vi "Main.vi"(10 "Tree Ref":refnum<vi>, 11 "Module Admin":refnum<class "Delacor_lib_QMH_Cloneable Module Admin.lvclass">) -> ()   [LabVIEW 2023, in "Tree Handlr.lvlib"]
doc: "This template is based off of the Queued Message Handler design pattern and the Queued Message Handler project template that ships with LabVIEW.\n\nThe main difference is that the queue is private to this module and communication between modules is performed via Broadcast and Request events.\n\nRequest events are wrapped in public API methods and are handled in the Event Handling Loop (EHL) of this VI. Any module can register for Broadcast events sent by this module. The EHL generates messages based on user interface actions.\n\nThe Message Handling Loop (MHL) processes messages generated by the EHL, or by other messages. The messages are string values, so new messages can be added easily to the Message Cases case structure in the MHL. Each message cluster can also provide an optional value for Message Data, which is a variant that can be converted to whatever message-specific data is required.\n_____\nBased on DQMH Project Template 7.0.1.1316."
uses:
  Tree Handlr.lvlib
  <vilib>/Delacor/Delacor QMH/Libraries/Cloneable Module Admin_class/Delacor_lib_QMH_Cloneable Module Admin.lvclass
  Module Data--cluster.ctl
  <vilib>/Delacor/Delacor QMH/Libraries/Message Queue_class/Delacor_lib_QMH_Message Queue.lvclass/Delacor_lib_QMH_Message Queue.ctl
  <vilib>/Delacor/Delacor QMH/Libraries/Cloneable Module Admin_class/Delacor_lib_QMH_Cloneable Module Admin.lvclass/Delacor_lib_QMH_Cloneable Module Admin.ctl
  Stop Argument--cluster.ctl
  <vilib>/Delacor/Delacor QMH/Libraries/Module Admin_class/Delacor_lib_QMH_Module Admin.lvclass/Delacor_lib_QMH_Module Admin.ctl
  Restore Open Items Argument--cluster.ctl
  <vilib>/Utility/miscctls.llb/LVPointTypeDef.ctl
  <vilib>/Delacor/Delacor QMH/Libraries/Message Queue_class/Delacor_lib_QMH_Enqueue Message (Multiline).vi
  <vilib>/Delacor/Delacor QMH/Libraries/Cloneable Module Admin_class/Delacor_lib_QMH_Get Module ID.vi
  <vilib>/Delacor/Delacor QMH/Libraries/Module Admin_class/Delacor_lib_QMH_Get External Launch.vi
  LabVIEW-common/TEMPLATES/State Machine/State Machine Sub/Process Multi-LineState String.vi
  <vilib>/Utility/inputDevices.llb/keyboardAcquire.vi
  <vilib>/Delacor/Delacor QMH/Libraries/Message Queue_class/Delacor_lib_QMH_Message Queue.lvclass
panel:
  out "error out":errorcluster
  out "Status":string
  in  "Simulate EHL Error":bool
  in  "Simulate MHL Error":bool
  # "Other processes communicate with this Module via its Public API (wrappers for its Request Events).\n\nThis Module communicates with other processes via its Broadcast Events.\nAny process that wants to receive these messages can register for this module's Broadcast events."
  # "This template is for the DQMH framework. See the block diagram for more information on how to use this template."
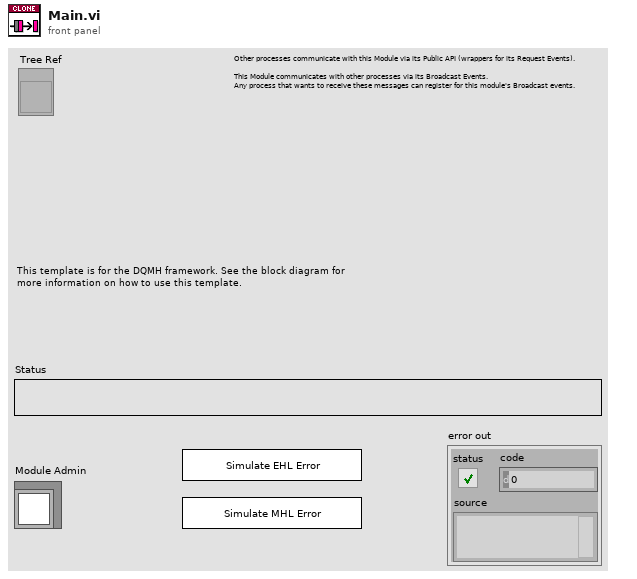
[diagram p1: front panel]
types:
  T1 = typedef "Tree Handlr.lvlib/Request Events--cluster.ctl" = cluster{"Stop Module":refnum<user-event>, "Show Panel":refnum<user-event>, "Hide Panel":refnum<user-event>, "Show Diagram":refnum<user-event>, "Get Module Execution Status":refnum<user-event>, "Restore Open Items":refnum<user-event>}
  T2 = typedef "Tree Handlr.lvlib/Module Data--cluster.ctl" = cluster{"Status":string}
  T3 = enum32{"invalid lock state", "Not Locked", "Locked (No Password)", "Password-protected"}
  T4 = typedef "Tree Handlr.lvlib/Stop Argument--cluster.ctl" = cluster{"Module ID":i32, "Origin":string, "Exit via Stop Module Req?":bool, "Wait for Module to stop?":bool}
  T5 = enum16{"0", "1", "2", "3", "4", "5", "6", "7", "8", "9", "A", "B", "C", "D", "E", "F", "G", "H", "I", "J", "K", "L", "M", "N", "O", "P", "Q", "R", "S", "T", "U", "V", "W", "X", "Y", "Z", "F1", "F2", "F3", "F4", "F5", "F6", "F7", "F8", "F9", "F10", "F11", "F12", "F13", "F14", "F15", "ADD", "BACK", "BACKSLASH", "CAPITAL", "COMMA", "DECIMAL", "DELETE", "DIVIDE", "DOWN", "END", "EQUALS", "ESCAPE", "GRAVE (`)", "HOME", "INSERT", "LBRACKET", "LCONTROL", "LEFT", "L ALT", "LSHIFT", "LWIN", "MINUS", "MULTIPLY", "NEXT", "NUMLOCK", "NUMPAD_0", "NUMPAD_1", "NUMPAD_2", "NUMPAD_3", "NUMPAD_4", "NUMPAD_5", "NUMPAD_6", "NUMPAD_7", "NUMPAD_8", "NUMPAD_9", "PAUSE", "PERIOD", "PRIOR (PG UP)", "RBRACKET", "RCONTROL", "RETURN", "RIGHT", "R ALT", "RSHIFT", "RWIN", "SCROLL", "SEMICOLON", "SLASH", "SPACE", "SUBTRACT", "TAB", "UP", "ENTER (num pad)", "' (quote)"}
  T6 = typedef "Tree Handlr.lvlib/Restore Open Items Argument--cluster.ctl" = cluster{"Module ID":i32, "Boolean":bool}
  T7 = typedef "LVPointTypeDef.ctl" = cluster{"Horizontal":i16, "Vertical":i16}
  T8 = enum32{"Invalid", "Standard", "Closed", "Hidden", "Minimized", "Maximized"}
  T9 = enum16{"0", "1", "2", "3", "4", "5", "6", "7", "8", "9", "A", "B", "C", "D", "E", "F", "G", "H", "I", "J", "K", "L", "M", "N", "O", "P", "Q", "R", "S", "T", "U", "V", "W", "X", "Y", "Z", "F1", "F2", "F3", "F4", "F5", "F6", "F7", "F8", "F9", "F10", "F11", "F12", "F13", "F14", "F15", "ADD", "BACK", "BACKSLASH", "CAPITAL", "COMMA", "DECIMAL", "DELETE", "DIVIDE", "DOWN", "END", "EQUALS", "ESCAPE", "GRAVE (`)", "HOME", "INSERT", "LBRACKET", "LCONTROL", "LEFT", "L ALT", "LSHIFT", "LWIN", "MINUS", "MULTIPLY", "NEXT", "NUMLOCK", "NUMPAD_0", "NUMPAD_1", "NUMPAD_2", "NUMPAD_3", "NUMPAD_4", "NUMPAD_5", "NUMPAD_6", "NUMPAD_7", "NUMPAD_8", "NUMPAD_9", "PAUSE", "PERIOD", "PRIOR (PG UP)", "RBRACKET", "RCONTROL", "RETURN", "RIGHT", "R ALT", "RSHIFT", "RWIN", "SCROLL", "SEMICOLON", "SLASH", "SPACE", "SUBTRACT", "TAB", "UP", "ENTER (num pad)", "' (quote)"}[]
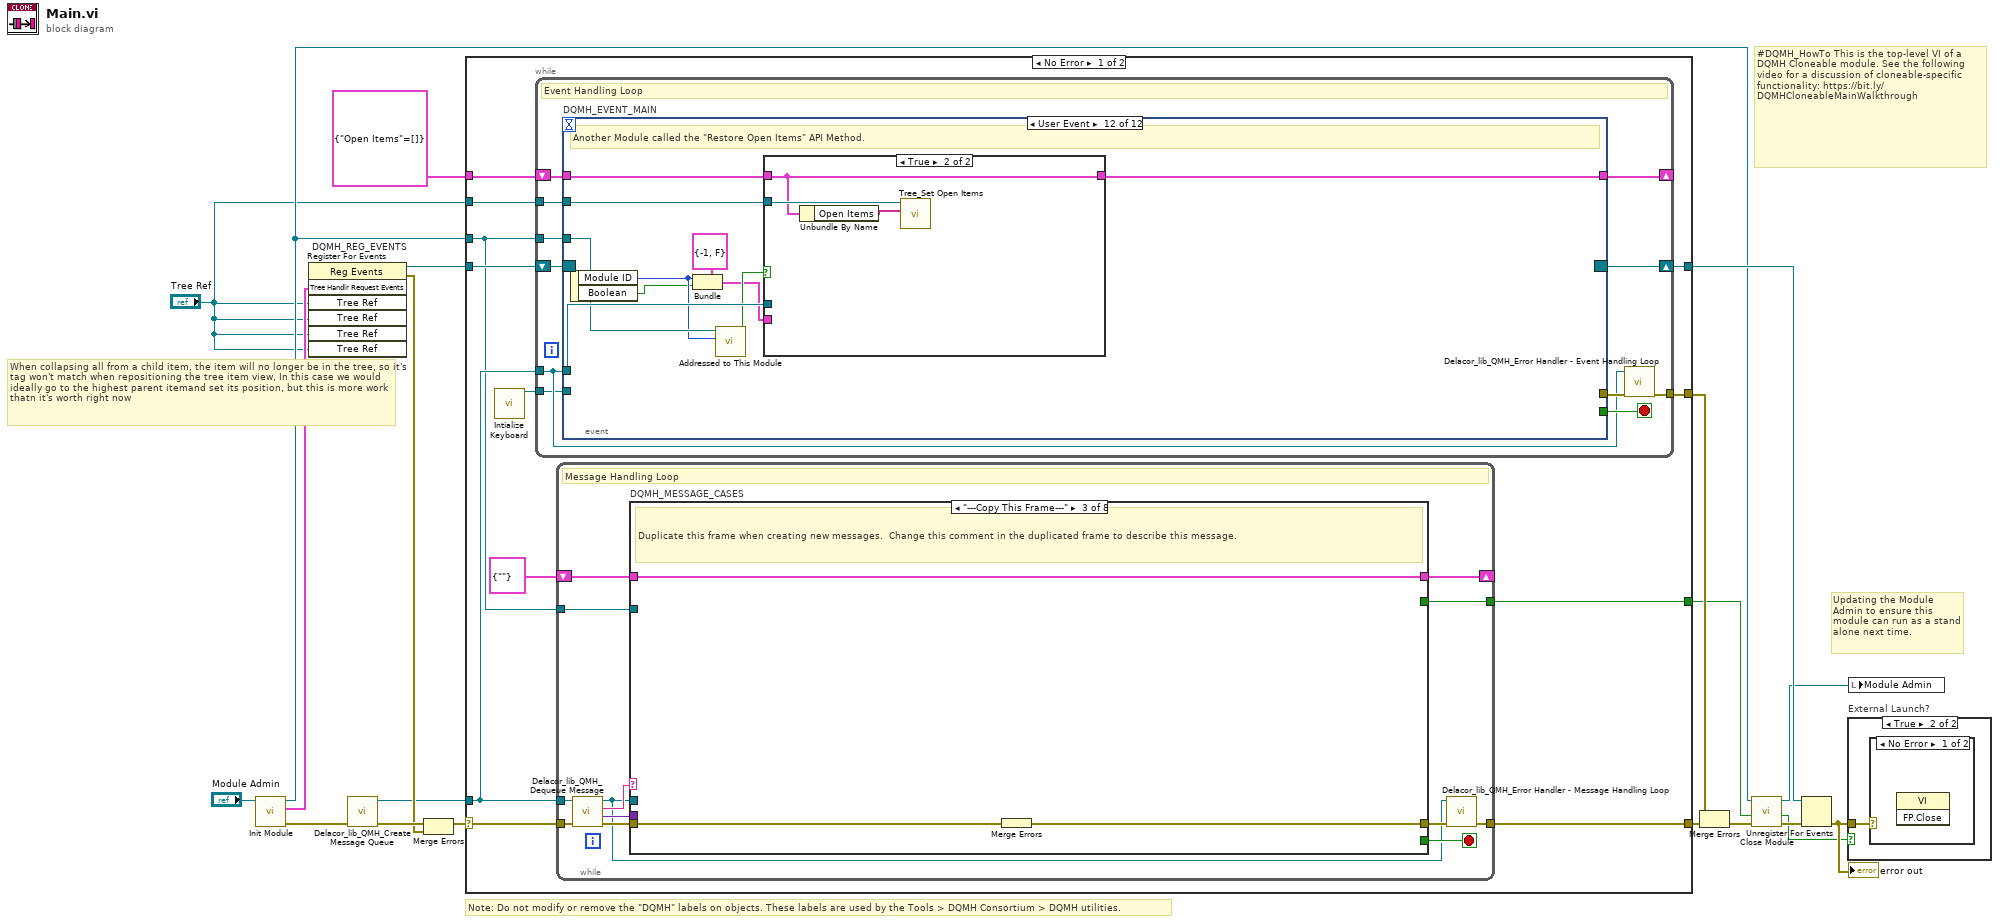
[diagram p0: block diagram]
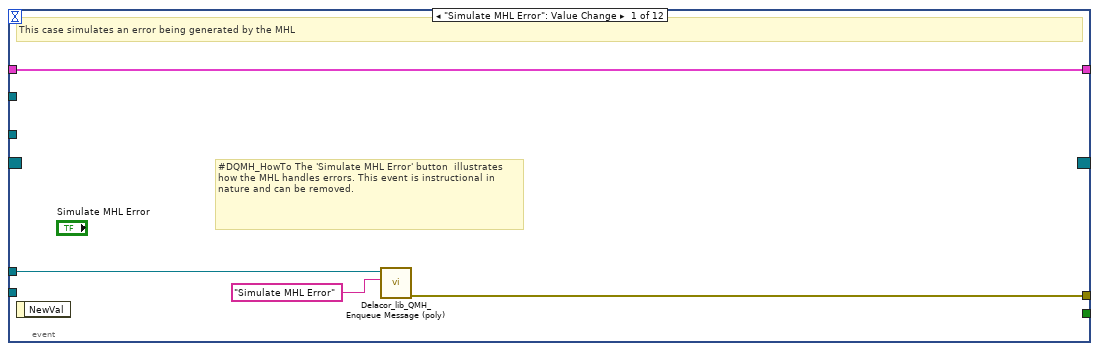
[diagram p2: hidden frame]
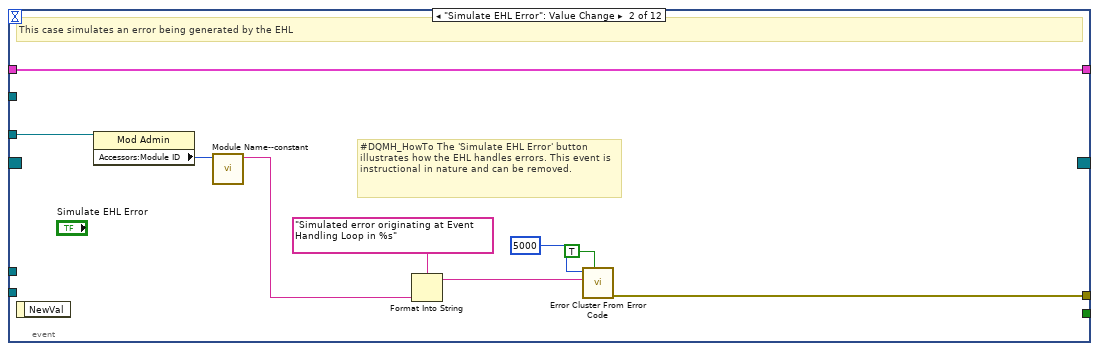
[diagram p3: hidden frame]
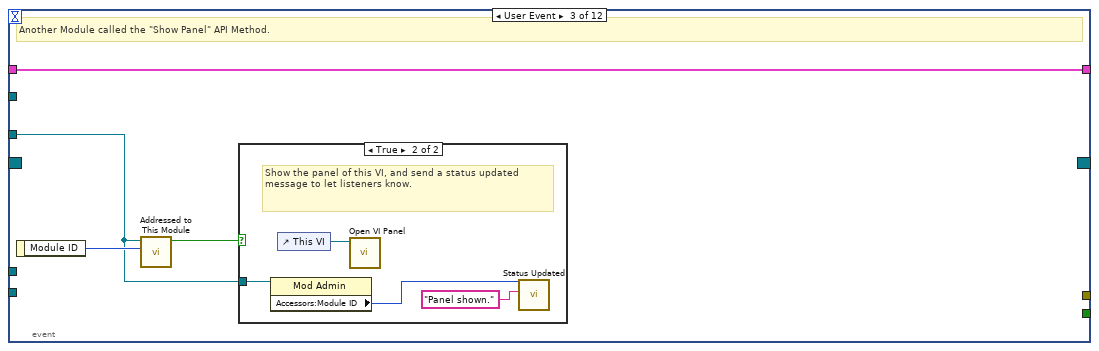
[diagram p4: hidden frame]
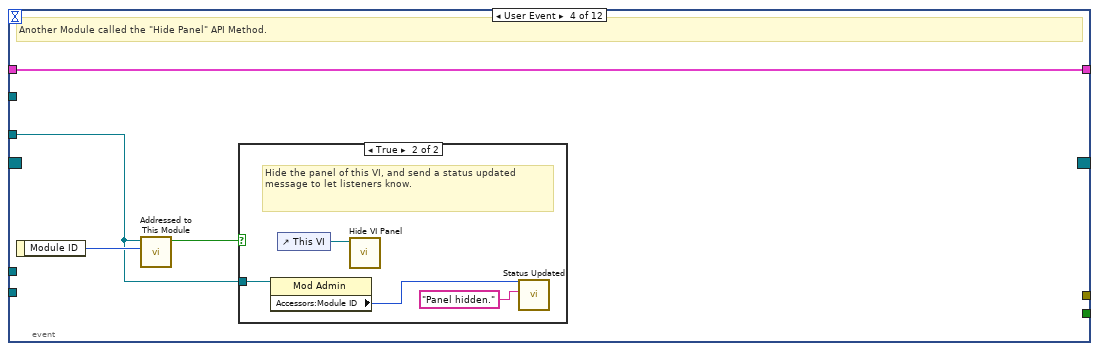
[diagram p6: hidden frame]
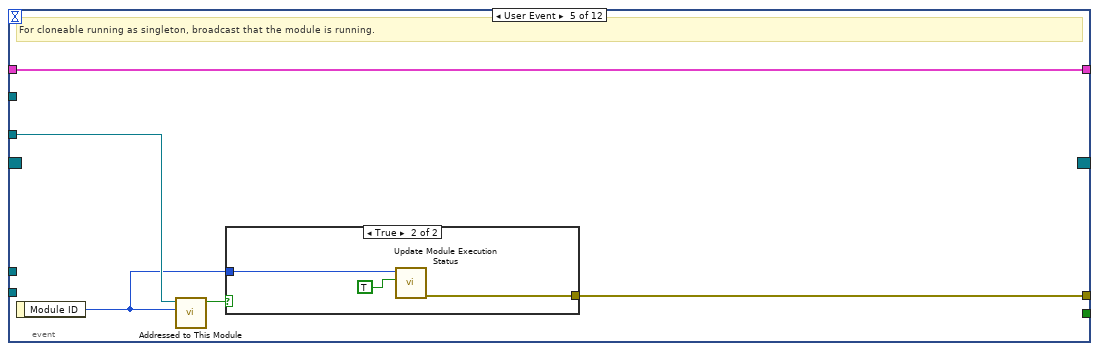
[diagram p8: hidden frame]
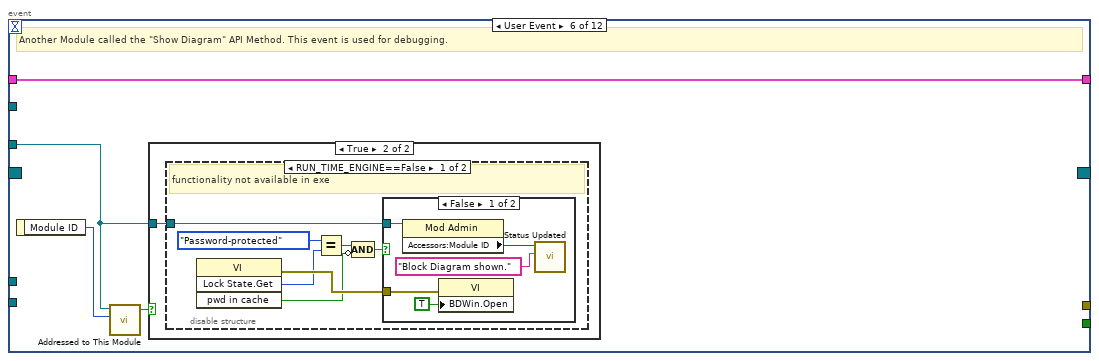
[diagram p10: hidden frame]
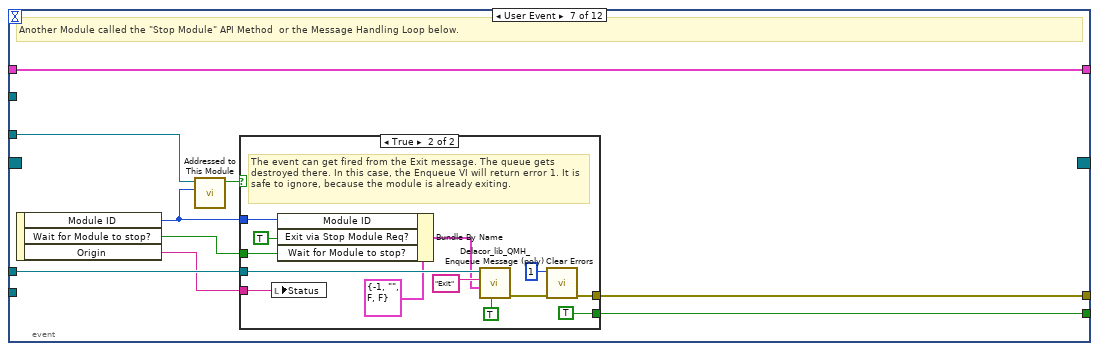
[diagram p14: hidden frame]
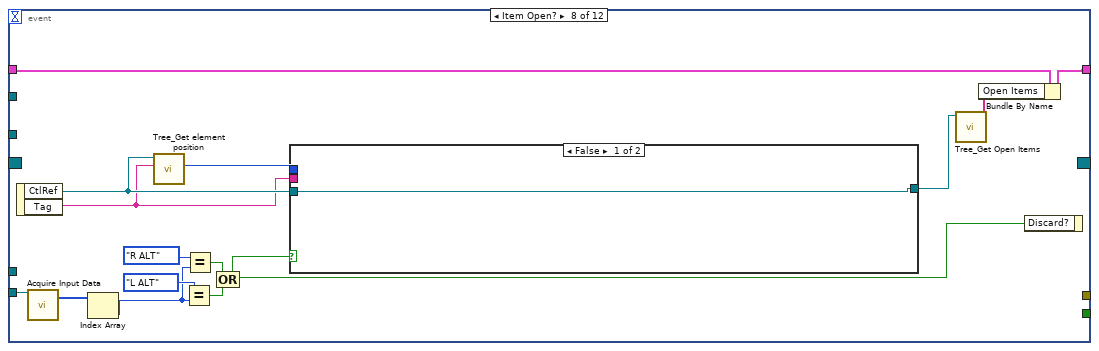
[diagram p16: hidden frame]
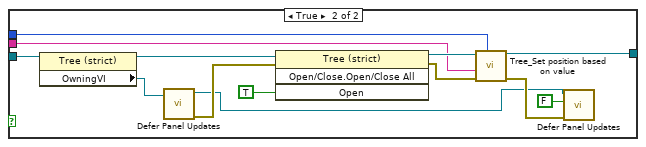
[diagram p17: hidden frame]
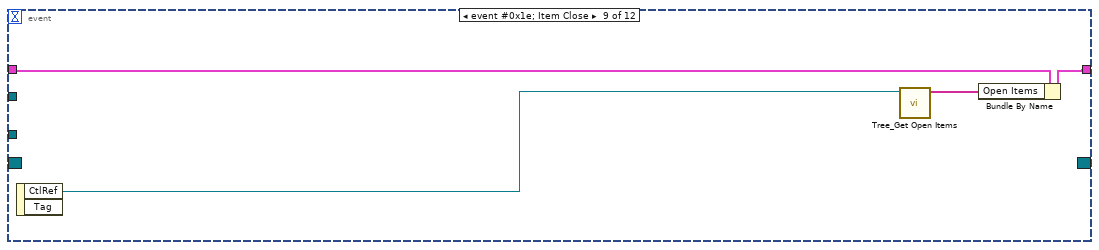
[diagram p18: hidden frame]
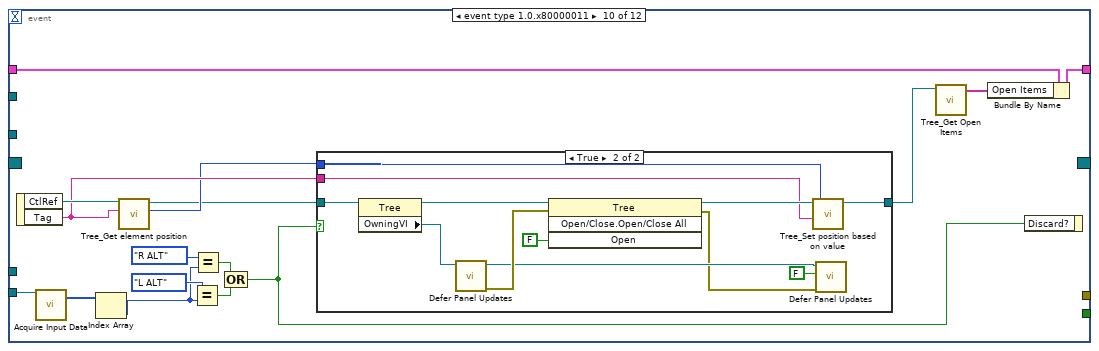
[diagram p19: hidden frame]
diagram:
  # "When collapsing all from a child item, the item will no longer be in the tree, so it's tag won't match when repositioning the tree item view, In this case we would ideally go to the highest parent itemand set its position, but this is more work thatn it's worth right now"
  # "#DQMH_HowTo This is the top-level VI of a DQMH Cloneable module. See the following video for a discussion of cloneable-specific functionality: https://bit.ly/DQMHCloneableMainWalkthrough"
  # "Note: Do not modify or remove the \"DQMH\" labels on objects. These labels are used by the Tools > DQMH Consortium > DQMH utilities."
  # "Updating the Module Admin to ensure this module can run as a stand alone next time."
  n1 = call "Init Module.vi"("Cloneable Module Admin in"="Module Admin") -> ("error out"=w17:errorcluster, "Tree Handlr Request Events"=w9:T1, "Cloneable Module Admin out"=w6:refnum<class "Delacor_lib_QMH_Cloneable Module Admin.lvclass">)  [unwired: 8 in]
  n2 = register-events "DQMH_REG_EVENTS"(w9, "Tree Ref", "Tree Ref", "Tree Ref", "Tree Ref") -> (reference out=w10:refnum<event-registration>, error out=w12:errorcluster)  [unwired: 2 in]
  n3 = call <vilib>:"Delacor_lib_QMH_Create Message Queue.vi"("error in"=w17) -> ("error out"=w14:errorcluster, "Message Queue"=w8:refnum<class "Delacor_lib_QMH_Message Queue.lvclass">)  [unwired: 9 in]
  n4 = Merge Errors(w14, w12) -> (w13:errorcluster)
  n5 = case shown="No Error" w13 {
    selector: w13 -> [w30 w320]
    tunnel: [w32 w319] -> w18
    tunnel: [w29 w318] -> w11
    tunnel: w10 -> [w27 w318]
    tunnel: w8 -> [w26 w311]
    tunnel: [w31 _] -> w19
    tunnel: w6 -> [w25 w314]
    tunnel: [w24 _] -> w4
    tunnel: cluster{"Open Items":string[]} {"Open Items"=[]} -> [w22 _]
    tunnel: "Tree Ref" -> [w21 _]
    frame No Error {
      n6 = call <vilib>:"Intialize Keyboard.vi"() -> ("device ID"=w23:refnum<k1>)  [unwired: 10 in, 1 out]
      n7 = while {
        tunnel: w26 -> [w37]
        shift-right: [w40] -> w29
        shift-left: w27 -> [w41]
        tunnel: [w42] -> w31
        tunnel: w25 -> [w38]
        tunnel: w23 -> [w36]
        shift-right: [w34] -> _
        shift-left: w22 -> [w35]
        tunnel: w21 -> [w33]
        stop <- w39 stop-if-true
        # "Event Handling Loop"
        n8 = event "DQMH_EVENT_MAIN" shown="[8] <Tree Ref>: Item Open;  <Tree Ref>: Item Close" {
          selector: w41 -> [_ _ _ _ _ _ _ _ _ _ _ _]
          dyn-events: [_ _ _ _ _ _ _ _ _ _ _ _] -> w40
          timeout: _ -> [_ _ _ _ _ _ _ _ _ _ _ _]
          tunnel: [_ _ _ _ _ _ w102 _ _ _ _ _] -> w39
          tunnel: w37 -> [w46 _ _ _ _ _ w105 _ _ _ w185 w207]
          tunnel: [w47 w56 _ _ w77 _ w106 _ _ _ w188 _] -> w43
          tunnel: w38 -> [_ w55 w58 w66 w75 w82 w104 _ _ _ w186 w205]
          tunnel: w36 -> [_ _ _ _ _ _ _ w128 _ w162 _ _]
          tunnel: w35 -> [w44 w48 w57 w65 w73 w81 w98 w123 w152 w157 w182 w199]
          tunnel: [w44 w48 w57 w65 w73 w81 w98 w122 w151 w156 w182 w198] -> w34
          tunnel: w33 -> [_ _ _ _ _ _ _ _ _ _ _ w200]
          event "Simulate MHL Error": Value Change {
            # "#DQMH_HowTo The 'Simulate MHL Error' button  illustrates how the MHL handles errors. This event is instructional in nature and can be removed."
            # "This case simulates an error being generated by the MHL"
            n9 = event-data() -> ()  [unwired: 1 in, 1 out]
            n10 = call-poly <vilib>:"Delacor_lib_QMH_Enqueue Message (poly).vi"("Message"="Simulate MHL Error", "Message Queue in"=w46) -> ("error out"=w47:errorcluster)  [unwired: 8 in, 1 out]
          }
          event "Simulate EHL Error": Value Change {
            # "#DQMH_HowTo The 'Simulate EHL Error' button  illustrates how the EHL handles errors. This event is instructional in nature and can be removed."
            # "This case simulates an error being generated by the EHL"
            n11 = event-data() -> ()  [unwired: 1 in, 1 out]
            n12 = property on="Property Node" class="Mod Admin"(reference=w55) -> ("Accessors:Module ID"=w54:i32)  [unwired: 1 in, 2 out]
            n13 = call "Module Name--constant.vi"("Module ID"=w54) -> ("Module Name"=w49:string)  [unwired: 10 in]
            n14 = Format Into String(format string="Simulated error originating at Event Handling Loop in %s", w49) -> (resulting string=w52:string)  [unwired: 2 in, 1 out]
            n15 = call <vilib>:"Error Cluster From Error Code.vi"("show call chain? (False)"=TRUE, "error message (\"\")"=w52, "error code (0)"=5000) -> ("error out"=w56:errorcluster)  [unwired: 6 in]
          }
          event User Event {
            # "Another Module called the \"Show Panel\" API Method."
            n16 = event-data() -> ("Module ID"=w59:i32)  [unwired: 1 in]
            n17 = call "Addressed to This Module.vi"("Module ID from Argument"=w59, "Module Admin"=w58) -> ("Addressed to this instance?"=w60:bool)  [unwired: 8 in, 1 out]
            n18 = case shown="True" w60 {
              tunnel: w58 -> [_ w62]
              frame False {
              }
              frame True {
                # "Show the panel of this VI, and send a status updated message to let listeners know."
                n19 = property on="Property Node" class="Mod Admin"(reference=w62) -> ("Accessors:Module ID"=w61:i32)  [unwired: 1 in, 2 out]
                n20 = control-ref of="This VI"() -> (w64:refnum<vi>)
                n21 = call "Open VI Panel.vi"("VI"=w64) -> ()  [unwired: 10 in, 1 out]
                n22 = call "Status Updated.vi"("Status"="Panel shown." ("format string"), "Module ID"=w61) -> ()  [unwired: 9 in, 1 out]
              }
            }
          }
          event User Event {
            # "Another Module called the \"Hide Panel\" API Method."
            n23 = event-data() -> ("Module ID"=w67:i32)  [unwired: 1 in]
            n24 = call "Addressed to This Module.vi"("Module ID from Argument"=w67, "Module Admin"=w66) -> ("Addressed to this instance?"=w68:bool)  [unwired: 8 in, 1 out]
            n25 = case shown="True" w68 {
              tunnel: w66 -> [_ w70]
              frame False {
              }
              frame True {
                # "Hide the panel of this VI, and send a status updated message to let listeners know."
                n26 = property on="Property Node" class="Mod Admin"(reference=w70) -> ("Accessors:Module ID"=w69:i32)  [unwired: 1 in, 2 out]
                n27 = control-ref of="This VI"() -> (w72:refnum<vi>)
                n28 = call "Hide VI Panel.vi"("VI"=w72) -> ()  [unwired: 10 in, 1 out]
                n29 = call "Status Updated.vi"("Status"="Panel hidden." ("format string"), "Module ID"=w69) -> ()  [unwired: 9 in, 1 out]
              }
            }
          }
          event User Event {
            # "For cloneable running as singleton, broadcast that the module is running."
            n30 = event-data() -> ("Module ID"=w74:i32)  [unwired: 1 in]
            n31 = call "Addressed to This Module.vi"("Module ID from Argument"=w74, "Module Admin"=w75) -> ("Addressed to this instance?"=w76:bool)  [unwired: 8 in, 1 out]
            n32 = case shown="True" w76 {
              tunnel: [_ w80] -> w77
              tunnel: w74 -> [_ w79]
              frame False {
              }
              frame True {
                n33 = call "Update Module Execution Status.vi"("Running?"=TRUE, "Module ID"=w79) -> ("error out"=w80:errorcluster)  [unwired: 9 in]
              }
            }
          }
          event User Event {
            # "Another Module called the \"Show Diagram\" API Method. This event is used for debugging."
            n34 = event-data() -> ("Module ID"=w83:i32)  [unwired: 1 in]
            n35 = call "Addressed to This Module.vi"("Module ID from Argument"=w83, "Module Admin"=w82) -> ("Addressed to this instance?"=w84:bool)  [unwired: 8 in, 1 out]
            n36 = case shown="True" w84 {
              tunnel: w82 -> [_ w85]
              frame False {
              }
              frame True {
                n37 = disable-structure shown="RUN_TIME_ENGINE==False" {
                  disable-tunnel: w85 -> [w86 _]
                  frame condition #0 (active) {
                    # "functionality not available in exe"
                    n38 = invoke on="Invoke Node" class="VI" method="Lock State.Get"() -> (error out=w92:errorcluster, "Get Lock State"=w91:T3, "pwd in cache"=w88:bool)  [unwired: 4 in, 1 out]
                    n39 = Equal?(x=T3."Password-protected", y=w91) -> (x = y?=w89:bool)
                    n40 = Compound Arithmetic op=AND(w89, invert w88) -> (w87:bool)
                    n41 = case shown="False" w87 {
                      tunnel: w92 -> [w97 _]
                      tunnel: w86 -> [w94 _]
                      frame False {
                        n42 = property on="Property Node" class="Mod Admin"(reference=w94) -> ("Accessors:Module ID"=w93:i32)  [unwired: 1 in, 2 out]
                        n43 = property on="Property Node" class="VI"(error in=w97, "BDWin.Open"=TRUE ("Block Diagram Window:Open")) -> ()  [unwired: 1 in, 2 out]
                        n44 = call "Status Updated.vi"("Status"="Block Diagram shown." ("format string"), "Module ID"=w93) -> ()  [unwired: 9 in, 1 out]
                      }
                      frame True {
                        # "Password-protected VI, and the password is not in the cache. Do not show the diagram."
                      }
                    }
                  }
                  frame condition #1 {
                  }
                }
              }
            }
          }
          event User Event {
            # "Another Module called the \"Stop Module\" API Method  or the Message Handling Loop below."
            n45 = event-data() -> ("Module ID"=w100:i32, "Wait for Module to stop?"=w101:bool, "Origin"=w99:string)  [unwired: 1 in]
            n46 = call "Addressed to This Module.vi"("Module ID from Argument"=w100, "Module Admin"=w104) -> ("Addressed to this instance?"=w103:bool)  [unwired: 8 in, 1 out]
            n47 = case shown="True" w103 {
              tunnel: [_ w118] -> w106
              tunnel: w105 -> [_ w114]
              tunnel: [_ TRUE] -> w102
              tunnel: w101 -> [_ w109]
              tunnel: w100 -> [_ w111]
              tunnel: w99 -> [_ w107]
              frame False {
              }
              frame True {
                # "The event can get fired from the Exit message. The queue gets destroyed there. In this case, the Enqueue VI will return error 1. It is safe to ignore, because the module is already exiting."
                n48 = local write "Status"(w107) -> ()
                n49 = Bundle By Name(cluster=T4 {"Module ID"=-1, "Origin"="", "Exit via Stop Module Req?"=FALSE, "Wait for Module to stop?"=FALSE} ("Stop Argument"), "Module ID"=w111, "Exit via Stop Module Req?"=TRUE, "Wait for Module to stop?"=w109) -> (w108:T4)
                n50 = call-poly <vilib>:"Delacor_lib_QMH_Enqueue Message (poly).vi"("Priority Message? (F)"=TRUE, "Message Data"=w108, "Message"="Exit", "Message Queue in"=w114) -> ("error out"=w119:errorcluster)  [unwired: 6 in, 1 out]
                n51 = call <vilib>:"Clear Errors.vi"("error in (no error)"=w119, "specific error code to clear (0: all)"=1) -> ("error out"=w118:errorcluster)  [unwired: 4 in, 1 out]
              }
            }
          }
          event Item Open? {
            n52 = event-data() -> ("CtlRef"=w126:refnum<vi>, "Tag"=w125:string)  [unwired: 1 in]
            n53 = call-poly <vilib>:"Acquire Input Data.vi"("device ID"=w128) -> ("keys pressed"=w134:T9)  [unwired: 16 in, 2 out]
            n54 = Index Array(array=w134) -> (element=w131:T5)  [unwired: 1 in]
            n55 = call "Tree_Get element position.vi"("tag"=w125, "Tree Ref In"=w126) -> ("Tree Item Row"=w124:i32)  [unwired: 7 in, 2 out]
            n56 = Equal?(x=T5."L ALT" ("element"), y=w131) -> (x = y?=w129:bool)
            n57 = Equal?(x=T5."R ALT" ("element"), y=w131) -> (x = y?=w130:bool)
            n58 = Compound Arithmetic op=OR(w130, w129) -> (w127:bool)
            n59 = case shown="False" w127 {
              tunnel: w125 -> [_ w146]
              tunnel: w126 -> [w135 w141]
              tunnel: w124 -> [_ w137]
              tunnel: [w135 w136] -> w120
              frame False {
              }
              frame True {
                n60 = property class="Tree (strict)"(reference=w141) -> (reference out=w139:refnum<vi>, "OwningVI"=w140:refnum<vi>)  [unwired: 1 in, 1 out]
                n61 = call "Defer Panel Updates.vi"("VI Ref"=w140) -> ("error out"=w144:errorcluster, "VI Ref Out"=w138:refnum<vi>)  [unwired: 9 in]
                n62 = invoke class="Tree (strict)" method="Open/Close.Open/Close All"(reference=w139, error in=w144, "Open"=TRUE ("Open?")) -> (reference out=w147:refnum<vi>, error out=w142:errorcluster)  [unwired: 1 in, 2 out]
                n63 = call "Tree_Set position based on value.vi"("Set Position [-1, in range]"=w137, "error in (no error)"=w142, "tag"=w146, "Tree Ref"=w147) -> ("error out"=w143:errorcluster, "Tree Ref"=w136:refnum<vi>)  [unwired: 6 in]
                n64 = call "Defer Panel Updates.vi"("error in (no error)"=w143, "Defer Panel Updates [T]"=FALSE, "VI Ref"=w138) -> ()  [unwired: 7 in, 2 out]
              }
            }
            n65 = call "Tree_Get Open Items.vi"("Tree Ref"=w120) -> ("Open Tree Item Tags"=w121:string[])  [unwired: 10 in]
            n66 = Bundle By Name(cluster=w123, "Open Items"=w121) -> (w122:cluster{"Open Items":string[]})
            n67 = event-data("Discard?"=w127) -> ()  [unwired: 1 in, 1 out]
          }
          event event #0x1e; Item Close {
            n68 = event-data() -> ("CtlRef"=w149:refnum<vi>)  [unwired: 1 in, 1 out]
            n69 = call "Tree_Get Open Items.vi"("Tree Ref"=w149) -> ("Open Tree Item Tags"=w150:string[])  [unwired: 10 in]
            n70 = Bundle By Name(cluster=w152, "Open Items"=w150) -> (w151:cluster{"Open Items":string[]})
          }
          event event type 1.0.x80000011 {
            n71 = event-data() -> ("CtlRef"=w160:refnum<vi>, "Tag"=w159:string)  [unwired: 1 in]
            n72 = call-poly <vilib>:"Acquire Input Data.vi"("device ID"=w162) -> ("keys pressed"=w168:T9)  [unwired: 16 in, 2 out]
            n73 = Index Array(array=w168) -> (element=w165:T5)  [unwired: 1 in]
            n74 = call "Tree_Get element position.vi"("tag"=w159, "Tree Ref In"=w160) -> ("Tree Item Row"=w158:i32, "Tree Ref Out"=w154:refnum<vi>)  [unwired: 7 in, 1 out]
            n75 = Equal?(x=T5."L ALT" ("element"), y=w165) -> (x = y?=w163:bool)
            n76 = Equal?(x=T5."R ALT" ("element"), y=w165) -> (x = y?=w164:bool)
            n77 = Compound Arithmetic op=OR(w164, w163) -> (w161:bool)
            n78 = case shown="True" w161 {
              tunnel: w159 -> [_ w175]
              tunnel: w158 -> [_ w174]
              tunnel: w154 -> [w169 w173]
              tunnel: [w169 w170] -> w153
              frame False {
              }
              frame True {
                n79 = property class="Tree"(reference=w173) -> (reference out=w172:refnum<vi>, "OwningVI"=w171:refnum<vi>)  [unwired: 1 in, 1 out]
                n80 = call "Defer Panel Updates.vi"("VI Ref"=w171) -> ("error out"=w179:errorcluster, "VI Ref Out"=w177:refnum<vi>)  [unwired: 9 in]
                n81 = invoke class="Tree" method="Open/Close.Open/Close All"(reference=w172, error in=w179, "Open"=FALSE ("Open?")) -> (reference out=w180:refnum<vi>, error out=w176:errorcluster)  [unwired: 1 in, 2 out]
                n82 = call "Tree_Set position based on value.vi"("Set Position [-1, in range]"=w174, "tag"=w175, "Tree Ref"=w180) -> ("Tree Ref"=w170:refnum<vi>)  [unwired: 7 in, 1 out]
                n83 = call "Defer Panel Updates.vi"("error in (no error)"=w176, "Defer Panel Updates [T]"=FALSE, "VI Ref"=w177) -> ()  [unwired: 7 in, 2 out]
              }
            }
            n84 = call "Tree_Get Open Items.vi"("Tree Ref"=w153) -> ("Open Tree Item Tags"=w155:string[])  [unwired: 10 in]
            n85 = Bundle By Name(cluster=w157, "Open Items"=w155) -> (w156:cluster{"Open Items":string[]})
            n86 = event-data("Discard?"=w161) -> ()  [unwired: 1 in, 1 out]
          }
          event Panel Close? {
            w187 = TRUE  # Discard the event, the MHL is responsible for closing and stopping this VI.
            # "Hide the panel or send the 'Exit' message if the user clicks the 'X' on the module main VI panel."
            n87 = event-data() -> ()  [unwired: 1 in, 1 out]
            n88 = property on="Property Node" class="Mod Admin"(reference=w186) -> (reference out=w183:refnum<class "Delacor_lib_QMH_Cloneable Module Admin.lvclass">, "Accessors:External Launch"=w184:bool)  [unwired: 1 in, 1 out]
            n89 = case shown="True" w184 {
              tunnel: w185 -> [_ w196]
              tunnel: [_ w197] -> w188
              tunnel: w183 -> [w191 _]
              frame True {
                # "If externally launched, clicking the 'X' hides the panel, but doesn't close it."
                n90 = property on="Property Node" class="Mod Admin"(reference=w191) -> ("Accessors:Module ID"=w190:i32)  [unwired: 1 in, 2 out]
                n91 = call "Status Updated.vi"("Status"="Panel hidden." ("format string"), "Module ID"=w190) -> ("error out"=w189:errorcluster)  [unwired: 9 in]
                n92 = control-ref of="This VI"() -> (w193:refnum<vi>)
                n93 = call "Hide VI Panel.vi"("error in"=w189, "VI"=w193) -> ()  [unwired: 9 in, 1 out]
              }
              frame False {
                # "If run as a stand-alone VI, clicking the panel 'X' stops the VI."
                n94 = call-poly <vilib>:"Delacor_lib_QMH_Enqueue Message (poly).vi"("Priority Message? (F)"=TRUE, "Message"="Exit", "Message Queue in"=w196) -> ("error out"=w197:errorcluster)  [unwired: 7 in, 1 out]
              }
            }
            n95 = event-data ("Event Filter Node")("Discard?"=w187) -> ()  [unwired: 1 in, 1 out]
          }
          event User Event {
            # "Another Module called the \"Restore Open Items\" API Method."
            n96 = event-data() -> ("Module ID"=w202:i32, "Boolean"=w201:bool)  [unwired: 1 in]
            n97 = Bundle(cluster=T6 {"Module ID"=-1, "Boolean"=FALSE} ("Restore Open Items Argument"), "Module ID"=w202, "Boolean"=w201) -> (w203:T6)
            n98 = call "Addressed to This Module.vi"("Module ID from Argument"=w202, "Module Admin"=w205) -> ("Addressed to this instance?"=w206:bool)  [unwired: 8 in, 1 out]
            n99 = case shown="True" w206 {
              tunnel: w207 -> [_ _]
              tunnel: w203 -> [_ _]
              tunnel: w200 -> [_ w211]
              tunnel: w199 -> [w208 w209]
              tunnel: [w208 w209] -> w198
              frame False {
              }
              frame True {
                n100 = Unbundle By Name(w209) -> ("Open Items"=w210:string[])
                n101 = call "Tree_Set Open Items.vi"("Open Tree Item Tags"=w210, "Tree Ref"=w211) -> ()  [unwired: 10 in]
              }
            }
          }
        }
        n102 = call-dynamic "Delacor_lib_QMH_Error Handler - Event Handling Loop.vi"("error in"=w43, "Message Queue in"=w37) -> ("dup error in"=w42:errorcluster)  [unwired: 8 in, 1 out]
      }
      n103 = while {
        tunnel: w26 -> [w212]
        shift-right: [w219] -> _
        shift-left: T2 {"Status"=""} ("Data Cluster") -> [w220]
        tunnel: w30 -> [w223]
        tunnel: [w221] -> w32
        tunnel: w25 -> [w214]
        tunnel: [w213] -> w24
        stop <- w218 stop-if-true
        # "Message Handling Loop"
        n104 = call-dynamic "Delacor_lib_QMH_Dequeue Message.vi"("error in"=w223, "Message Queue in"=w212) -> ("error out"=w222:errorcluster, "Message Data"=w216:variant, "Message"=w217:string, "Message Queue out"=w215:refnum<class "Delacor_lib_QMH_Message Queue.lvclass">)  [unwired: 6 in]
        n105 = case "DQMH_MESSAGE_CASES" shown="\"---Copy This Frame---\"" w217 {
          selector: w217 -> [_ _ _ _ _ _ _ w300]
          tunnel: w215 -> [_ _ _ _ w255 _ w292 _]
          tunnel: w222 -> [w243 w247 w250 w252 w264 w281 w298 w309]
          tunnel: [w241 w247 w249 w252 w260 w280 w293 w310] -> w224
          tunnel: w220 -> [w234 w246 w248 w251 w259 w278 w291 w307]
          tunnel: [w233 w246 w248 w251 w259 w278 w291 w307] -> w219
          tunnel: [_ _ _ _ _ _ w290 _] -> w218
          tunnel: w216 -> [_ _ _ _ w258 _ w288 _]
          tunnel: w214 -> [w228 _ _ _ w257 w276 w283 w306]
          tunnel: [_ _ _ _ _ _ w286 _] -> w213
          frame "Initialize" {
            w225 = "Initial Message" ("Initial Message")
            # "#CodeNeeded - Initialize the appearance of the front panel."
            # "#CodeNeeded - Initialize your state data here."
            # "Initialize - Any operation that needs to be done before the module can receive messages. Synchronize Caller Events.vi will inform Start Module.vi that the module has launched and is ready to receive messages. Module Did Init.vi will broadcast that the module initialized."
            n106 = call "Synchronize Caller Events.vi"("error in"=w243, "Module Admin"=w228) -> ("error out"=w242:errorcluster, "Module Admin out"=w227:refnum<class "Delacor_lib_QMH_Cloneable Module Admin.lvclass">)  [unwired: 8 in]
            n107 = property on="Property Node" class="Mod Admin"(reference=w227) -> ("Accessors:Module ID"=w230:i32, "Accessors:External Launch"=w229:bool)  [unwired: 1 in, 2 out]
            n108 = call "Module Name--constant.vi"("Module ID"=w230) -> ("Module Name"=w238:string)  [unwired: 10 in]
            n109 = property on="Property Node" class="VI"("Front Panel.Title"=w238) -> (reference out=w240:refnum<vi>, error out=w245:errorcluster)  [unwired: 2 in]
            n110 = Select(t=T8."Hidden" ("State"), s=w229, f=T8."Standard" ("State")) -> (s? t:f=w235:T8)
            n111 = invoke on="Invoke Node" class="VI" method="FP.Open"(reference=w240, error in=w245, "State"=w235) -> (reference out=w239:refnum<vi>, error out=w244:errorcluster)  [unwired: 2 in, 3 out]
            n112 = call "Module Name--constant.vi"("Module ID"=w230) -> ("Module Name"=w231:string)  [unwired: 10 in]
            n113 = Bundle By Name(cluster=w234, "Status"=w225) -> (w233:T2)
            n114 = invoke on="Invoke Node" class="VI" method="FP.Center"(reference=w239, error in=w244) -> ()  [unwired: 1 in, 3 out]
            n115 = property on="Pane" class="Pane"("Origin"=T7 {"Horizontal"=0, "Vertical"=0}) -> ()  [unwired: 2 in, 2 out]
            n116 = call "Module Did Init.vi"("error in"=w242, "Initialized?"=TRUE, "Origin"=w231, "Module ID"=w230) -> ("error out"=w241:errorcluster)  [unwired: 7 in]
            "Status" <- w225
          }
          frame "---Module Specific---" {
            # "Separator -- The following cases handle messages specific to this Module."
          }
          frame "---Copy This Frame---" {
            # "Duplicate this frame when creating new messages.  Change this comment in the duplicated frame to describe this message."
            n117 = Merge Errors(w250) -> (w249:errorcluster)
          }
          frame "---Exit and Error Handling---" {
            # "Separator - the following cases handle errors and exit messages."
          }
          frame "Error" {
            # "#CodeRecommended - If the module is running in standalone mode (External Launch = FALSE), this code will pop up an error dialog and call the 'Exit' message if an error occurs. Add more fine-grained error management here."
            # "Error - Check the error message data and respond accordingly. This message is sent by the \"Error Handler\" VIs at the end of each loop in this application."
            n118 = property on="Property Node" class="Mod Admin"(reference=w257) -> ("Accessors:External Launch"=w256:bool, "Accessors:Module ID"=w254:i32)  [unwired: 1 in, 2 out]
            n119 = Variant To Data(error in=w264, type=errorcluster {"status"=FALSE, "code"=0, "source"=""} ("error constant"), Variant=w258) -> (data=w253:errorcluster, error out=w262:errorcluster)
            n120 = local write "error out"(w253) -> ()
            n121 = call "Error Reported.vi"("Error"=w253, "Module ID"=w254) -> ()  [unwired: 9 in, 1 out]
            n122 = case shown="False" w256 {
              tunnel: [w269 _] -> w261
              tunnel: w255 -> [w267 _]
              tunnel: w253 -> [w268 _]
              frame False {
                n123 = disable-structure shown="Default" {
                  disable-tunnel: w268 -> [w270 _]
                  frame condition #0 (active) {
                    # "If the module is running standalone, then pop up an error dialog and call the \"Exit\" message."
                    n124 = call <vilib>:"Simple Error Handler.vi"("error in (no error)"=w270) -> ()  [unwired: 4 in, 5 out]
                  }
                  frame condition #1 {
                    # "To prevent the Simple Error Handler VI from being loaded (e.g. when deploying to a Real-Time target), add the Conditional Disable Symbol \"DQMH_Disable_SEH\" to your project and set it to TRUE."
                  }
                }
                n125 = call-poly <vilib>:"Delacor_lib_QMH_Enqueue Message (poly).vi"("Priority Message? (F)"=TRUE, "Message"="Exit", "Message Queue in"=w267) -> ("error out"=w269:errorcluster)  [unwired: 7 in, 1 out]
              }
              frame True {
                # "If the module was launched externally, calling the Error Reported broadcast VI is the only action performed by the \"Error\" message. The module's caller can then process the error appropriately."
              }
            }
            n126 = Merge Errors(w262, w261) -> (w260:errorcluster)
          }
          frame "Simulate MHL Error" {
            # "#DQMH_HowTo The 'Simulate MHL Error' button  illustrates how the MHL handles errors. This event is instructional in nature and can be removed."
            # "Simulate an error occurring at the MHL"
            n127 = property on="Property Node" class="Mod Admin"(reference=w276) -> ("Accessors:Module ID"=w277:i32)  [unwired: 1 in, 2 out]
            n128 = call "Module Name--constant.vi"("Module ID"=w277) -> ("Module Name"=w272:string)  [unwired: 10 in]
            n129 = Format Into String(format string="Simulated error originating at Message Handling Loop in %s", w272) -> (resulting string=w273:string)  [unwired: 2 in, 1 out]
            n130 = call <vilib>:"Error Cluster From Error Code.vi"("show call chain? (False)"=TRUE, "error message (\"\")"=w273, "error code (0)"=5001) -> ("error out"=w279:errorcluster)  [unwired: 6 in]
            n131 = Merge Errors(w281, w279) -> (w280:errorcluster)
          }
          frame "Exit" {
            w289 = 91  # 91: not all Exit messages will have an argument
            w290 = TRUE  # Stop the VI
            # "Release the message queue reference"
            # "#CodeNeeded - Add any required cleanup code here."
            # "Exit - Exit the application."
            n132 = Variant To Data(error in=w298, type=T4 {"Module ID"=-1, "Origin"="", "Exit via Stop Module Req?"=FALSE, "Wait for Module to stop?"=FALSE} ("Stop Argument"), Variant=w288) -> (data=w285:T4, error out=w294:errorcluster)
            n133 = call <vilib>:"Clear Errors.vi"("error in (no error)"=w294, "specific error code to clear (0: all)"=w289) -> ("error out"=w297:errorcluster)  [unwired: 4 in, 1 out]
            n134 = property on="Property Node" class="Mod Admin"(reference=w283) -> ("Accessors:Module ID"=w282:i32)  [unwired: 1 in, 2 out]
            n135 = control-ref of="This VI"() -> (w284:refnum<vi>)
            n136 = call-dynamic "Delacor_lib_QMH_Release Message Queue.vi"("error in"=w297, "Message Queue"=w292) -> ("error out"=w296:errorcluster)  [unwired: 9 in]
            n137 = call "Handle Exit.vi"("Stop Argument"=w285, "Module Admin in"=w283, "VI reference"=w284) -> ("error out"=w295:errorcluster, "Wait for Stop?"=w286:bool)  [unwired: 7 in]
            n138 = Merge Errors(w296, w295) -> (w293:errorcluster)
            n139 = call "Error Reported.vi"("Error"=w293, "Module ID"=w282) -> ()  [unwired: 9 in, 1 out]
          }
          frame Default {
            # "'Default' case only runs if there is a message that isn't defined in any of the other cases.  Output a programming error."
            n140 = property on="Property Node" class="Mod Admin"(reference=w306) -> ("Accessors:Module ID"=w305:i32)  [unwired: 1 in, 2 out]
            n141 = call "Module Name--constant.vi"("Module ID"=w305) -> ("Module Name"=w299:string)  [unwired: 10 in]
            n142 = Format Into String(format string="The invalid message string \"%s\" was received in the Message Handling Loop for module \"%s\".", w300, w299) -> (resulting string=w302:string)  [unwired: 2 in, 1 out]
            n143 = call <vilib>:"Error Cluster From Error Code.vi"("show call chain? (False)"=TRUE, "error message (\"\")"=w302, "error code (0)"=1) -> ("error out"=w308:errorcluster)  [unwired: 6 in]
            n144 = Merge Errors(w309, w308) -> (w310:errorcluster)
          }
        }
        n145 = call-dynamic "Delacor_lib_QMH_Error Handler - Message Handling Loop.vi"("error in"=w224, "Message Queue in"=w215) -> ("dup error in"=w221:errorcluster)  [unwired: 8 in, 1 out]
      }
    }
    frame Error {
      n146 = call "Synchronize Caller Events.vi"("Module Admin"=w314) -> ("Module Admin out"=w313:refnum<class "Delacor_lib_QMH_Cloneable Module Admin.lvclass">)  [unwired: 9 in, 1 out]
      n147 = property on="Property Node" class="Mod Admin"(reference=w313) -> ("Accessors:Module ID"=w312:i32)  [unwired: 1 in, 2 out]
      n148 = call-dynamic "Delacor_lib_QMH_Release Message Queue.vi"("error in"=w320, "Message Queue"=w311) -> ("error out"=w319:errorcluster)  [unwired: 9 in]
      n149 = call "Module Name--constant.vi"("Module ID"=w312) -> ("Module Name"=w317:string)  [unwired: 10 in]
      n150 = Format Into String(format string="An error occurred during initialization. %s is no longer running.", w317) -> (resulting string=w315:string)  [unwired: 2 in, 1 out]
      n151 = call "Error Reported.vi"("Additional Information"=w315, "Error"=w319, "Module ID"=w312) -> ()  [unwired: 8 in, 1 out]
    }
  }
  n152 = Merge Errors(w19, w18) -> (w20:errorcluster)
  n153 = call "Close Module.vi"("error in"=w20, "Wait for stop?"=w4, "Module Admin in"=w6) -> ("error out"=w16:errorcluster, "External Launch"=w3:bool, "Module Admin out"=w5:refnum<class "Delacor_lib_QMH_Cloneable Module Admin.lvclass">)  [unwired: 6 in]
  n154 = Unregister For Events(event registration refnum=w11, error in=w16) -> (error out=w15:errorcluster)
  "error out" <- w15
  n155 = case "External Launch?" shown="True" w3 {
    tunnel: w15 -> [_ w321]
    frame False {
    }
    frame True {
      n156 = case shown="No Error" w321 {
        frame No Error {
          n157 = invoke class="VI" method="FP.Close"() -> ()  [unwired: 3 in, 3 out]
        }
        frame Error {
          n158 = invoke class="VI" method="FP.Open"("Activate"=TRUE ("Activate?")) -> ()  [unwired: 4 in, 5 out]
        }
      }
    }
  }
  n159 = local write "Module Admin"(w5) -> ()
